vi "Initialization VI.vi"(8 "error in (no error)":errorcluster, 10 "Custom XML":string, 11 "Device Item Ref in":T1 format="%.0x") -> (0 "error out":errorcluster, 3 "Device Item Ref out":T1 format="%.0x")   [LabVIEW 2016, in "DMM-SWITCH-ScanList System Explorer.lvlib"]
uses:
  DMM-SWITCH-ScanList System Explorer.lvlib
  <vilib>/NI Veristand/Custom Device API/Custom Device Item Ref.ctl
  <instrlib>/niDMM/nidmm.llb/niDMM Function.ctl
  <instrlib>/niDMM/nidmm.llb/niDMM Resolution in Digits.ctl
  <instrlib>/niSwitch/niSwitch.llb/niSwitch Topologies.ctl
  <instrlib>/niSwitch/niSwitch.llb/niSwitch Trigger Input.ctl
  <instrlib>/niSwitch/niSwitch.llb/niSwitch Scan Advanced Output.ctl
  <instrlib>/niDMM/nidmm.llb/niDMM Measurement Complete.ctl
  <instrlib>/niDMM/nidmm.llb/niDMM Trigger.ctl
  Pages/Configuration Controls/DMM Temp.ctl
  <instrlib>/niDMM/nidmm.llb/niDMM Transducer Type.ctl
  <instrlib>/niDMM/nidmm.llb/niDMM Thermocouple Type.ctl
  <instrlib>/niDMM/nidmm.llb/niDMM RTD Type.ctl
  <instrlib>/niDMM/nidmm.llb/niDMM Thermistor Type.ctl
  <vilib>/NI Veristand/Custom Device API/Custom Device Channel.ctl
  <vilib>/NI Veristand/Custom Device API/Custom Device Channel Type.ctl
  Shared/Constants.vi
  <vilib>/NI Veristand/Custom Device API/Custom Device API.lvlib
  Shared/DMM-SWITCH-ScanList Shared.lvlib
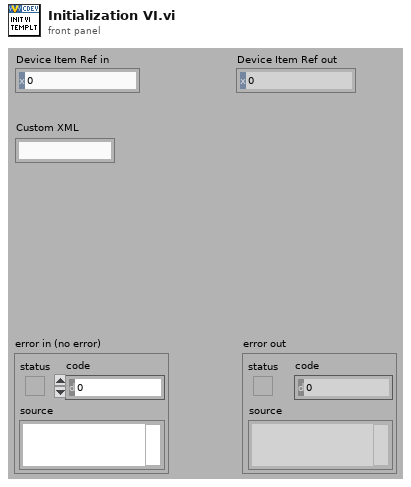
[diagram p1: front panel]
types:
  T1 = typedef "Custom Device API.lvlib/Custom Device Item Ref.ctl" = u64
  T2 = typedef "DMM-SWITCH-ScanList System Explorer.lvlib/DMM Temp.ctl" = cluster{"DMM Temp - Transducer Type":T3, "DMM Temp - Thermocouple Type":T4, "DMM Temp - Fixed Reference Junction":dbl, "DMM Temp - RTD Type":T5, "DMM Temp - RTD Resistance":dbl, "DMM Temp - Thermistor Type":T6, "DMM Temp - RTD A":dbl, "DMM Temp - RTD B":dbl, "DMM Temp - RTD C":dbl, "DMM Temp - Thermistor A":dbl, "DMM Temp - Thermistor B":dbl, "DMM Temp - Thermistor C":dbl}
  T3 = typedef "niDMM Transducer Type.ctl" = i32
  T4 = typedef "niDMM Thermocouple Type.ctl" = i32
  T5 = typedef "niDMM RTD Type.ctl" = enum16{"Custom", "Pt3750", "Pt3851", "Pt3911", "Pt3916", "Pt3920", "Pt3928"}
  T6 = typedef "niDMM Thermistor Type.ctl" = enum16{"Custom", "44004", "44006", "44007"}
  T7 = typedef "niDMM Trigger.ctl" = enum16{"Immediate", "External", "TTL 0", "TTL 1", "TTL 2", "TTL 3", "TTL 4", "TTL 5", "TTL 6", "Software", "TTL 7", "PXI Star", "LBR Trig 1", "Aux Trig 1"}
  T8 = typedef "niDMM Measurement Complete.ctl" = enum16{"None", "External", "TTL 0", "TTL 1", "TTL 2", "TTL 3", "TTL 4", "TTL 5", "TTL 6", "TTL 7", "LBR Trig 0"}
  T9 = typedef "niSwitch Scan Advanced Output.ctl" = enum16{"None", "External", "TTL0", "TTL1", "TTL2", "TTL3", "TTL4", "TTL5", "TTL6", "TTL7", "ECL0", "ECL1", "PXI Star", "Rear Connector", "Front Connector", "Rear Connector Module 1", "Rear Connector Module 2", "Rear Connector Module 3", "Rear Connector Module 4", "Rear Connector Module 5", "Rear Connector Module 6", "Rear Connector Module 7", "Rear Connector Module 8", "Rear Connector Module 9", "Rear Connector Module 10", "Rear Connector Module 11", "Rear Connector Module 12", "Front Connector Module 1", "Front Connector Module 2", "Front Connector Module 3", "Front Connector Module 4", "Front Connector Module 5", "Front Connector Module 6", "Front Connector Module 7", "Front Connector Module 8", "Front Connector Module 9", "Front Connector Module 10", "Front Connector Module 11", "Front Connector Module 12"}
  T10 = typedef "niSwitch Trigger Input.ctl" = enum16{"Immediate", "External", "TTL0", "TTL1", "TTL2", "TTL3", "TTL4", "TTL5", "TTL6", "TTL7", "ECL0", "ECL1", "PXI Star", "Software Trigger Function", "Rear Connector", "Front Connector", "Rear Connector of Module 1", "Rear Connector of Module 2", "Rear Connector of Module 3", "Rear Connector of Module 4", "Rear Connector of Module 5", "Rear Connector of Module 6", "Rear Connector of Module 7", "Rear Connector of Module 8", "Rear Connector of Module 9", "Rear Connector of Module 10", "Rear Connector of Module 11", "Rear Connector of Module 12", "Front Connector of Module 1", "Front Connector of Module 2", "Front Connector of Module 3", "Front Connector of Module 4", "Front Connector of Module 5", "Front Connector of Module 6", "Front Connector of Module 7", "Front Connector of Module 8", "Front Connector of Module 9", "Front Connector of Module 10", "Front Connector of Module 11", "Front Connector of Module 12"}
  T11 = typedef "niDMM Function.ctl" = enum16{"DC Volts", "AC Volts", "DC Current", "AC Current", "2-wire Resistance", "4-wire Resistance", "Diode", "Frequency", "Period", "AC Volts DC Coupled", "Capacitance", "Inductance", "Temperature"}
  T12 = typedef "niSwitch Topologies.ctl" = string
  T13 = typedef "niDMM Resolution in Digits.ctl" = dbl
  T14 = typedef "Custom Device API.lvlib/Custom Device Channel.ctl" = cluster{"Type":T15, "Units":string, "Default Value":dbl, "Faultable":bool, "Scalable":bool}
  T15 = typedef "Custom Device API.lvlib/Custom Device Channel Type.ctl" = enum16{"Input", "Output"}
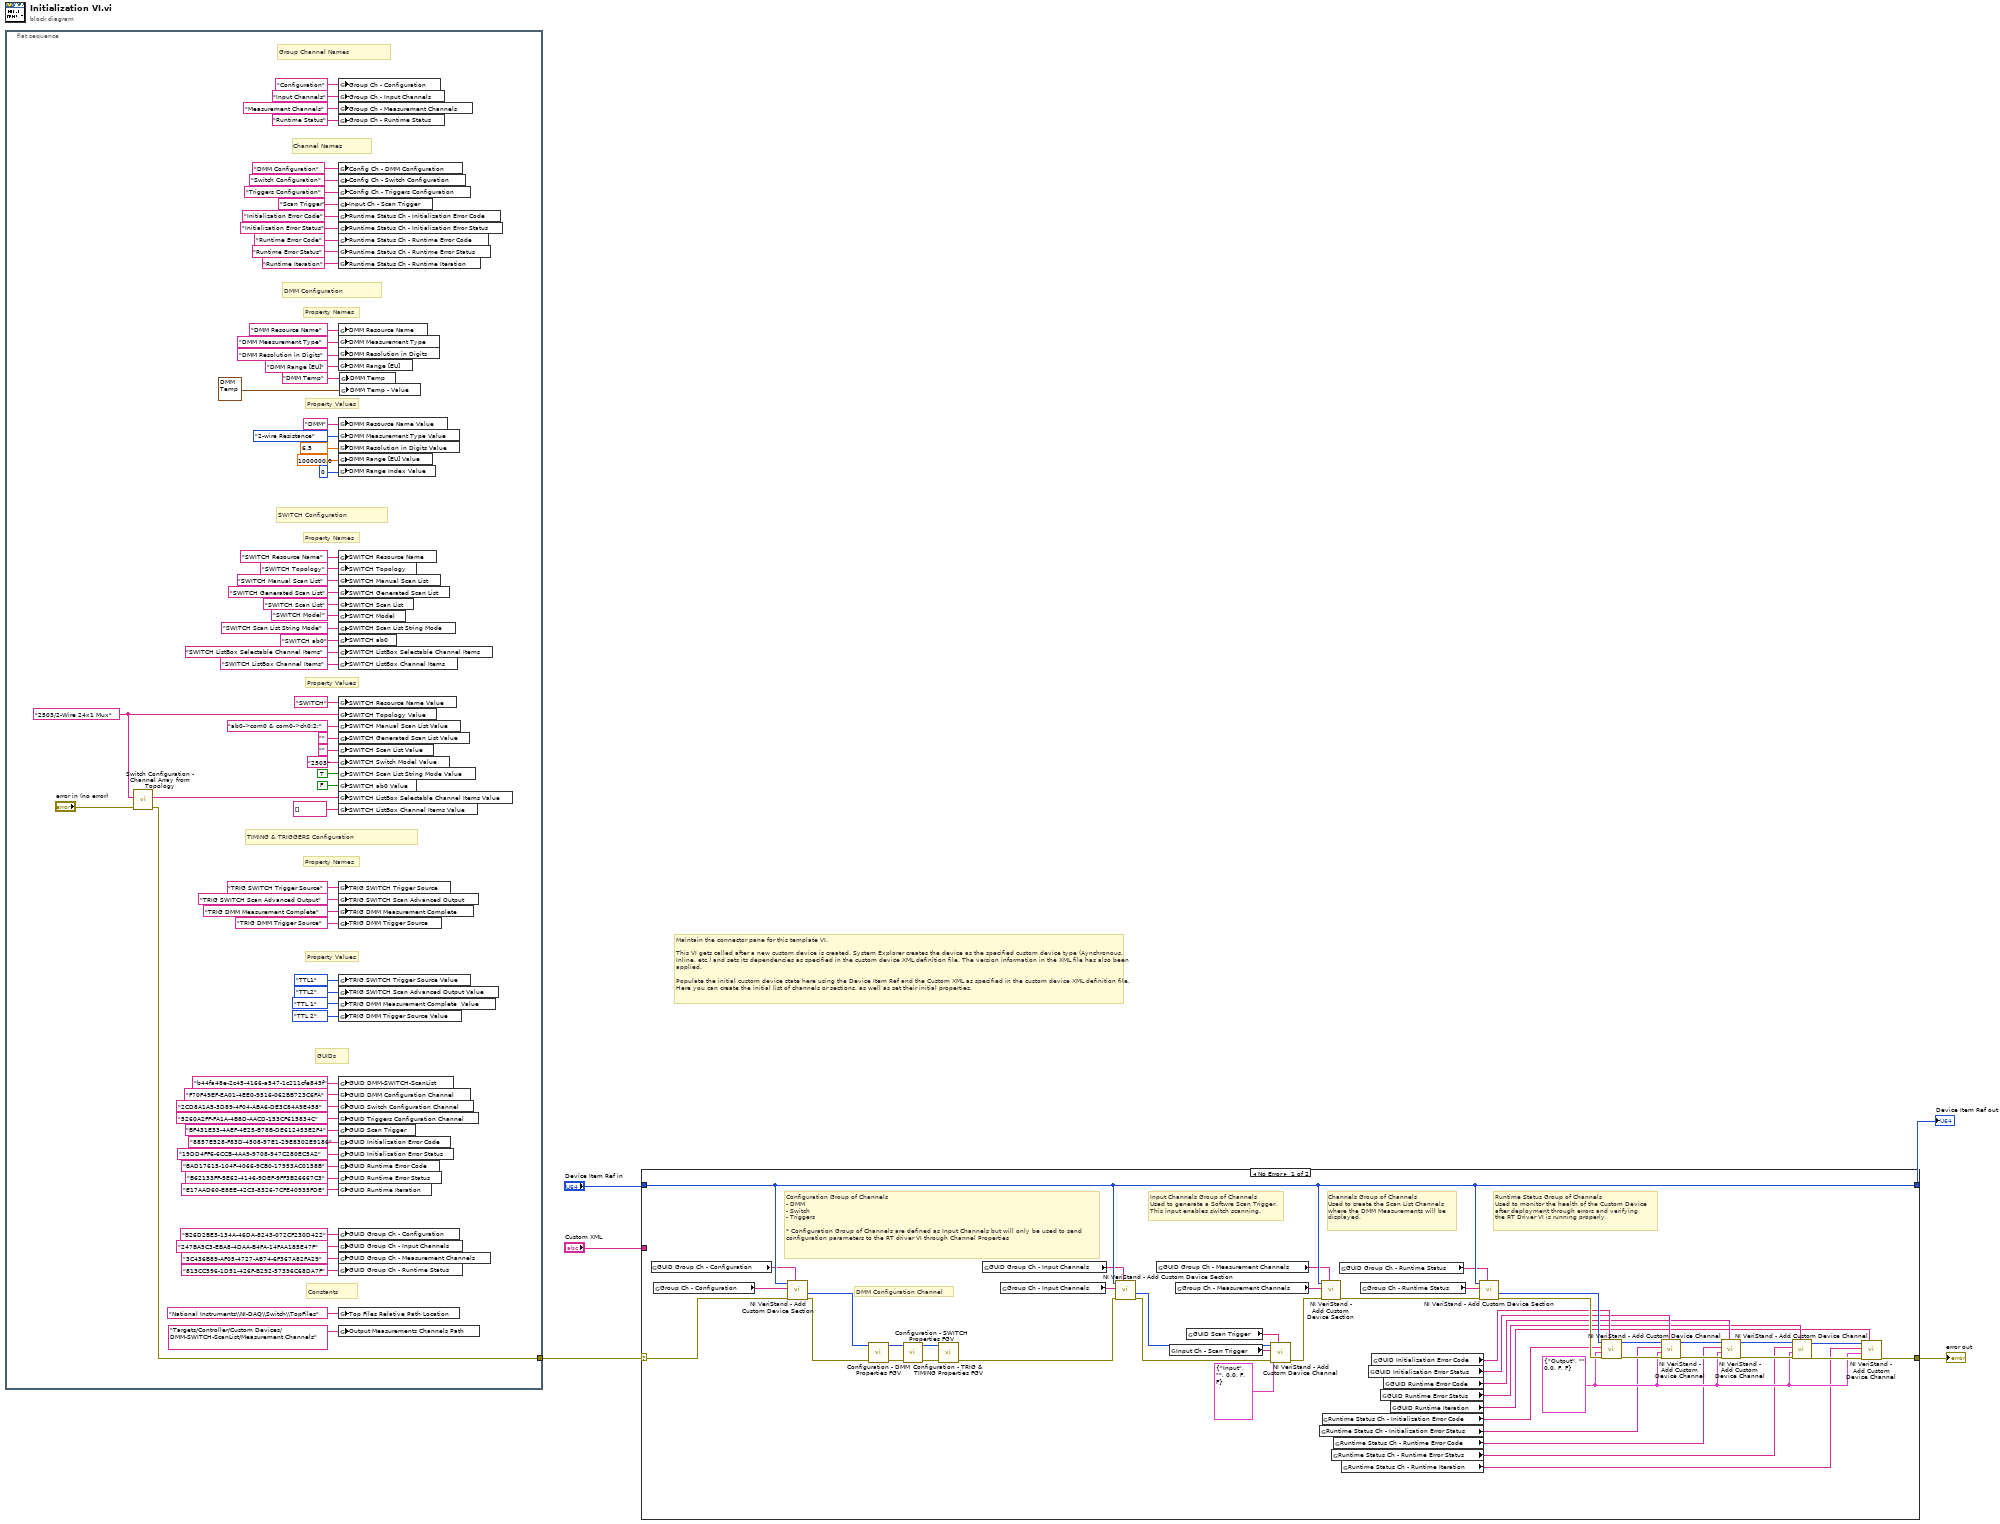
[diagram p0: block diagram]
diagram:
  # "Maintain the connector pane for this template VI.\n\nThis VI gets called after a new custom device is created. System Explorer creates the device as the specified custom device type (Aynchronous, Inline, etc.) and sets its dependencies as specified in the custom device XML definition file. The version information in the XML file has also been applied.\n\nPopulate the initial custom device state here using the Device Item Ref and the Custom XML as specified in the custom device XML definition file. Here you can create the initial list of channels or sections, as well as set their initial properties."
  n1 = flat-sequence {
    tunnel: [w56] -> w5
    frame #0 {
      w57 = T12 "2503/2-Wire 24x1 Mux" ("SWITCH Topology")
      w73 = T13 6.5 items=["3 1/2"=3.5, "4 1/2"=4.5, "5 1/2"=5.5, "6 1/2"=6.5, "7 1/2"=7.5] ("Resolution in Digits")
      # "Channel Names"
      # "Group Channel Names"
      # "Property Values"
      # "Property Names"
      # "Property Values"
      # "Property Names"
      # "Property Values"
      # "Property Names"
      # "Constants"
      # "DMM Configuration"
      # "GUIDs"
      # "TIMING & TRIGGERS Configuration"
      # "SWITCH Configuration"
      n2 = call "Switch Configuration - Channel Array from Topology.vi"("error in (no error)"="error in (no error)", "Selected Mux Topology"=w57) -> ("error out"=w56:errorcluster, "Channel Array Out"=w55:string[])  [unwired: 8 in]
      n3 = global write "Constants.vi" "Group Ch - Configuration"("Configuration" ("Group Ch - Configuration")) -> ()
      n4 = global write "Constants.vi" "Group Ch - Input Channels"("Input Channels" ("Group Ch - Input Channels")) -> ()
      n5 = global write "Constants.vi" "Group Ch - Measurement Channels"("Measurement Channels" ("Group Ch - Measurement Channels")) -> ()
      n6 = global write "Constants.vi" "Group Ch - Runtime Status"("Runtime Status" ("Group Ch - Runtime Status")) -> ()
      n7 = global write "Constants.vi" "Config Ch - DMM Configuration"("DMM Configuration" ("Group Ch - Configuration")) -> ()
      n8 = global write "Constants.vi" "Config Ch - Switch Configuration"("Switch Configuration" ("Group Ch - Input Channels")) -> ()
      n9 = global write "Constants.vi" "Config Ch - Triggers Configuration"("Triggers Configuration" ("Group Ch - Measurement Channels")) -> ()
      n10 = global write "Constants.vi" "Input Ch - Scan Trigger"("Scan Trigger" ("Group Ch - Runtime Status")) -> ()
      n11 = global write "Constants.vi" "Runtime Status Ch - Initialization Error Code"("Initialization Error Code" ("Group Ch - Configuration")) -> ()
      n12 = global write "Constants.vi" "Runtime Status Ch - Initialization Error Status"("Initialization Error Status" ("Group Ch - Input Channels")) -> ()
      n13 = global write "Constants.vi" "Runtime Status Ch - Runtime Error Code"("Runtime Error Code" ("Group Ch - Measurement Channels")) -> ()
      n14 = global write "Constants.vi" "Runtime Status Ch - Runtime Error Status"("Runtime Error Status" ("Group Ch - Runtime Status")) -> ()
      n15 = global write "Constants.vi" "Runtime Status Ch - Runtime Iteration"("Runtime Iteration" ("Group Ch - Runtime Status")) -> ()
      n16 = global write "Constants.vi" "DMM Resource Name"("DMM Resource Name" ("DMM Resource Name")) -> ()
      n17 = global write "Constants.vi" "DMM Measurement Type"("DMM Measurement Type" ("DMM Measurement Type")) -> ()
      n18 = global write "Constants.vi" "DMM Resolution in Digits"("DMM Resolution in Digits" ("DMM Resolution in Digits")) -> ()
      n19 = global write "Constants.vi" "DMM Range [EU]"("DMM Range [EU]" ("DMM Range [EU]")) -> ()
      n20 = global write "Constants.vi" "DMM Resource Name Value"("DMM" ("Value")) -> ()
      n21 = global write "Constants.vi" "DMM Measurement Type Value"(niDMM_Function."2-wire Resistance" ("Function")) -> ()
      n22 = global write "Constants.vi" "DMM Resolution in Digits Value"(w73) -> ()
      n23 = global write "Constants.vi" "DMM Range [EU] Value"(1000000.0 ("DMM Range [EU] Value")) -> ()
      n24 = global write "Constants.vi" "DMM Range Index Value"(u16 0 ("DMM Range Index")) -> ()
      n25 = global write "Constants.vi" "SWITCH Resource Name"("SWITCH Resource Name" ("SWITCH Resource Name")) -> ()
      n26 = global write "Constants.vi" "SWITCH Topology"("SWITCH Topology" ("SWITCH Topology")) -> ()
      n27 = global write "Constants.vi" "SWITCH Manual Scan List"("SWITCH Manual Scan List" ("SWITCH Manual Scan List")) -> ()
      n28 = global write "Constants.vi" "SWITCH Generated Scan List"("SWITCH Generated Scan List" ("SWITCH Generated Scan List")) -> ()
      n29 = global write "Constants.vi" "SWITCH Scan List"("SWITCH Scan List" ("SWITCH Scan List")) -> ()
      n30 = global write "Constants.vi" "SWITCH Model"("SWITCH Model" ("SWITCH Switch Model")) -> ()
      n31 = global write "Constants.vi" "SWITCH Scan List String Mode"("SWITCH Scan List String Mode" ("SWITCH Scan List String Mode")) -> ()
      n32 = global write "Constants.vi" "SWITCH ab0"("SWITCH ab0" ("SWITCH ab0")) -> ()
      n33 = global write "Constants.vi" "SWITCH ListBox Selectable Channel Items"("SWITCH ListBox Selectable Channel Items" ("SWITCH ListBox Selectable Channel Items")) -> ()
      n34 = global write "Constants.vi" "SWITCH ListBox Channel Items"("SWITCH ListBox Channel Items" ("SWITCH ListBox Channel Items")) -> ()
      n35 = global write "Constants.vi" "SWITCH Resource Name Value"("SWITCH" ("SWITCH Resource Name")) -> ()
      n36 = global write "Constants.vi" "SWITCH Topology Value"(w57) -> ()
      n37 = global write "Constants.vi" "SWITCH Manual Scan List Value"("ab0->com0 & com0->ch0:2;" ("SWITCH Manual Scan List")) -> ()
      n38 = global write "Constants.vi" "SWITCH Generated Scan List Value"("" ("SWITCH Generated Scan List")) -> ()
      n39 = global write "Constants.vi" "SWITCH Scan List Value"("" ("SWITCH Scan List")) -> ()
      n40 = global write "Constants.vi" "SWITCH Switch Model Value"("2503" ("SWITCH Switch Model")) -> ()
      n41 = global write "Constants.vi" "SWITCH Scan List String Mode Value"(TRUE ("SWITCH Scan List String Mode")) -> ()
      n42 = global write "Constants.vi" "SWITCH ab0 Value"(FALSE ("SWITCH ab0")) -> ()
      n43 = global write "Constants.vi" "SWITCH ListBox Selectable Channel Items Value"(w55) -> ()
      n44 = global write "Constants.vi" "SWITCH ListBox Channel Items Value"(string[] [] ("SWITCH ListBox Channel Items")) -> ()
      n45 = global write "Constants.vi" "TRIG SWITCH Trigger Source"("TRIG SWITCH Trigger Source" ("TRIG SWITCH Trigger Source")) -> ()
      n46 = global write "Constants.vi" "TRIG SWITCH Scan Advanced Output"("TRIG SWITCH Scan Advanced Output" ("TRIG SWITCH Scan Advanced Output")) -> ()
      n47 = global write "Constants.vi" "TRIG DMM Measurement Complete"("TRIG DMM Measurement Complete" ("TRIG DMM Measurement Complete")) -> ()
      n48 = global write "Constants.vi" "TRIG DMM Trigger Source"("TRIG DMM Trigger Source" ("TRIG DMM Trigger Source")) -> ()
      n49 = global write "Constants.vi" "TRIG SWITCH Trigger Source Value"(niSwitch_Trigger_Input."TTL1" ("TRIG SWITCH Trigger Source")) -> ()
      n50 = global write "Constants.vi" "TRIG SWITCH Scan Advanced Output Value"(niSwitch_Scan_Advanced_Output."TTL2" ("TRIG SWITCH Scan \nAdvanced Output")) -> ()
      n51 = global write "Constants.vi" "TRIG DMM Measurement Complete  Value"(niDMM_Measurement_Complete."TTL 1" ("TRIG DMM Measurement \nComplete Destination")) -> ()
      n52 = global write "Constants.vi" "TRIG DMM Trigger Source Value"(niDMM_Trigger."TTL 2" ("TRIG DMM Trigger Source")) -> ()
      n53 = global write "Constants.vi" "GUID DMM-SWITCH-ScanList"("b44fa48e-2c45-4166-a547-1c211cfe843f" ("GUID DMM-SWITCH-ScanList")) -> ()
      n54 = global write "Constants.vi" "GUID DMM Configuration Channel"("F70F49EF-EA01-4EE0-9516-062BB723C6FA" ("GUID DMM Configuration Channel")) -> ()
      n55 = global write "Constants.vi" "GUID Switch Configuration Channel"("2CD8A1A5-3D89-4F04-ABA6-DE3C84A9E458" ("GUID Switch Configuration Channel")) -> ()
      n56 = global write "Constants.vi" "GUID Triggers Configuration Channel"("5260A2FF-FA1A-4B8D-AACD-153CF615834C" ("GUID Triggers Configuration Channel")) -> ()
      n57 = global write "Constants.vi" "GUID Scan Trigger"("BF431E33-4AEF-4E25-B78B-DE612453E2F4" ("GUID DMM-SWITCH-ScanList")) -> ()
      n58 = global write "Constants.vi" "GUID Initialization Error Code"("8857E528-F83D-4508-97E1-29E8302E9186" ("GUID DMM Configuration Channel")) -> ()
      n59 = global write "Constants.vi" "GUID Initialization Error Status"("19DD4FF6-6CCB-4AA9-9708-947C280EC5A2" ("GUID Switch Configuration Channel")) -> ()
      n60 = global write "Constants.vi" "GUID Runtime Error Code"("BAD17615-104F-4066-9CB0-17953AC0158B" ("GUID Triggers Configuration Channel")) -> ()
      n61 = global write "Constants.vi" "GUID Runtime Error Status"("B62133FF-5E62-4146-9DEF-9FF3B26667C3" ("GUID Triggers Configuration Channel")) -> ()
      n62 = global write "Constants.vi" "GUID Runtime Iteration"("E17AAD60-E8EE-42C3-8326-7CFE40935FDE" ("GUID Triggers Configuration Channel")) -> ()
      n63 = global write "Constants.vi" "GUID Group Ch - Configuration"("B26D2BE3-134A-46DA-8243-072CF230D422" ("GUID Triggers Configuration Channel")) -> ()
      n64 = global write "Constants.vi" "GUID Group Ch - Input Channels"("247BA5C3-EBA8-4DAA-B4FA-14FAA185E47F" ("GUID Triggers Configuration Channel")) -> ()
      n65 = global write "Constants.vi" "GUID Group Ch - Measurement Channels"("3C436B89-AF05-4727-AB74-6F367A82FA29" ("GUID Triggers Configuration Channel")) -> ()
      n66 = global write "Constants.vi" "GUID Group Ch - Runtime Status"("813CC596-1D51-426F-B292-57396C68DA7F" ("GUID Triggers Configuration Channel")) -> ()
      n67 = global write "Constants.vi" "Top Files Relative Path Location"("National Instruments\\NI-DAQ\\Switch\\TopFiles" ("Top Files Relative Path Location")) -> ()
      n68 = global write "Constants.vi" "Output Measurements Channels Path"("Targets/Controller/Custom Devices/DMM-SWITCH-ScanList/Measurement Channels" ("Output Measurements Channels Path")) -> ()
      n69 = global write "Constants.vi" "DMM Temp"("DMM Temp" ("DMM Temp")) -> ()
      n70 = global write "Constants.vi" "DMM Temp - Value"(T2 {"DMM Temp - Transducer Type"=1, "DMM Temp - Thermocouple Type"=6, "DMM Temp - Fixed Reference Junction"=25.0, "DMM Temp - RTD Type"=enum."Pt3851", "DMM Temp - RTD Resistance"=100.0, "DMM Temp - Thermistor Type"=enum."44006", "DMM Temp - RTD A"=0.0039083, "DMM Temp - RTD B"=-5.775e-07, "DMM Temp - RTD C"=-4.183e-12, "DMM Temp - Thermistor A"=0.0010295, "DMM Temp - Thermistor B"=0.0002391, "DMM Temp - Thermistor C"=1.568e-07} ("DMM Temp - Value")) -> ()
    }
  }
  n71 = case shown="No Error" w5 {
    selector: w5 -> [w117 w123]
    tunnel: [w93 w123] -> w1
    tunnel: [w98 w122] -> w3
    tunnel: "Device Item Ref in" -> [w98 w122]
    tunnel: "Custom XML" -> [_ _]
    frame No Error {
      w104 = T14 {"Type"=enum."Output", "Units"="", "Default Value"=0.0, "Faultable"=FALSE, "Scalable"=FALSE} ("Channel")
      # "Input Channels Group of Channels\nUsed to generate a Softwre Scan Trigger.\nThis input enables switch scanning."
      # "Runtime Status Group of Channels\nUsed to monitor the health of the Custom Device\nafter deployment through errors and verifying \nthe RT Driver VI is running properly."
      # "Channels Group of Channels\nUsed to create the Scan List Channels\nwhere the DMM Measurements will be\ndisplayed."
      # "DMM Configuration Channel"
      # "Configuration Group of Channels\n- DMM\n- Switch\n- Triggers\n\n* Configuration Group of Channels are defined as Input Channels but will only be used to send \nconfiguration parameters to the RT driver VI through Channel Properties"
      n72 = global read "Constants.vi" "GUID Group Ch - Configuration"() -> (w85:string)
      n73 = global read "Constants.vi" "Group Ch - Configuration"() -> (w86:string)
      n74 = call <vilib>:"NI VeriStand - Add Custom Device Section.vi"("GUID (Default Section)"=w85, "error in (no error)"=w117, "Section Name"=w86, "Parent Ref in"=w98) -> ("error out"=w121:errorcluster, "Section Ptr"=w120:T1)  [unwired: 4 in, 2 out]
      n75 = call "Configuration - DMM Properties FGV.vi"("error in (no error)"=w121, "Configuration Group of Channels Ref In"=w120) -> ("error out"=w116:errorcluster, "Configuration Group of Channels Ref Out"=w119:T1)  [unwired: 8 in]
      n76 = call "Configuration - SWITCH Properties FGV.vi"("error in (no error)"=w116, "Parent Ref in"=w119) -> ("error out"=w115:errorcluster, "Parent Ref out"=w118:T1)  [unwired: 8 in]
      n77 = call "Configuration - TRIG & TIMING Properties FGV.vi"("error in (no error)"=w115, "Parent Ref in"=w118) -> ("error out"=w100:errorcluster)  [unwired: 9 in]
      n78 = global read "Constants.vi" "GUID Group Ch - Input Channels"() -> (w84:string)
      n79 = global read "Constants.vi" "Group Ch - Input Channels"() -> (w96:string)
      n80 = call <vilib>:"NI VeriStand - Add Custom Device Section.vi"("GUID (Default Section)"=w84, "error in (no error)"=w100, "Section Name"=w96, "Parent Ref in"=w98) -> ("error out"=w102:errorcluster, "Section Ptr"=w103:T1)  [unwired: 4 in, 2 out]
      n81 = global read "Constants.vi" "GUID Group Ch - Measurement Channels"() -> (w83:string)
      n82 = global read "Constants.vi" "Input Ch - Scan Trigger"() -> (w92:string)
      n83 = global read "Constants.vi" "Group Ch - Measurement Channels"() -> (w95:string)
      n84 = global read "Constants.vi" "GUID Scan Trigger"() -> (w76:string)
      n85 = call <vilib>:"NI VeriStand - Add Custom Device Channel.vi"("GUID (Default Channel)"=w76, "error in (no error)"=w102, "Channel"=T14 {"Type"=enum."Input", "Units"="", "Default Value"=0.0, "Faultable"=FALSE, "Scalable"=FALSE}, "Channel Name"=w92, "Parent Ref in"=w103) -> ("error out"=w101:errorcluster)  [unwired: 3 in, 3 out]
      n86 = global read "Constants.vi" "Runtime Status Ch - Initialization Error Status"() -> (w90:string)
      n87 = call <vilib>:"NI VeriStand - Add Custom Device Section.vi"("GUID (Default Section)"=w83, "error in (no error)"=w101, "Section Name"=w95, "Parent Ref in"=w98) -> ("error out"=w114:errorcluster)  [unwired: 4 in, 3 out]
      n88 = global read "Constants.vi" "Runtime Status Ch - Initialization Error Code"() -> (w91:string)
      n89 = global read "Constants.vi" "Runtime Status Ch - Runtime Error Status"() -> (w88:string)
      n90 = global read "Constants.vi" "Runtime Status Ch - Runtime Error Code"() -> (w89:string)
      n91 = global read "Constants.vi" "GUID Group Ch - Runtime Status"() -> (w82:string)
      n92 = global read "Constants.vi" "Runtime Status Ch - Runtime Iteration"() -> (w87:string)
      n93 = global read "Constants.vi" "Group Ch - Runtime Status"() -> (w94:string)
      n94 = global read "Constants.vi" "GUID Initialization Error Status"() -> (w80:string)
      n95 = global read "Constants.vi" "GUID Initialization Error Code"() -> (w81:string)
      n96 = global read "Constants.vi" "GUID Runtime Error Status"() -> (w78:string)
      n97 = global read "Constants.vi" "GUID Runtime Error Code"() -> (w79:string)
      n98 = global read "Constants.vi" "GUID Runtime Iteration"() -> (w77:string)
      n99 = call <vilib>:"NI VeriStand - Add Custom Device Section.vi"("GUID (Default Section)"=w82, "error in (no error)"=w114, "Section Name"=w94, "Parent Ref in"=w98) -> ("error out"=w106:errorcluster, "Section Ptr"=w105:T1)  [unwired: 4 in, 2 out]
      n100 = call <vilib>:"NI VeriStand - Add Custom Device Channel.vi"("GUID (Default Channel)"=w81, "error in (no error)"=w106, "Channel"=w104, "Channel Name"=w91, "Parent Ref in"=w105) -> ("error out"=w113:errorcluster, "Parent Ref out"=w97:T1)  [unwired: 3 in, 2 out]
      n101 = call <vilib>:"NI VeriStand - Add Custom Device Channel.vi"("GUID (Default Channel)"=w80, "error in (no error)"=w113, "Channel"=w104, "Channel Name"=w90, "Parent Ref in"=w97) -> ("error out"=w111:errorcluster, "Parent Ref out"=w112:T1)  [unwired: 3 in, 2 out]
      n102 = call <vilib>:"NI VeriStand - Add Custom Device Channel.vi"("GUID (Default Channel)"=w79, "error in (no error)"=w111, "Channel"=w104, "Channel Name"=w89, "Parent Ref in"=w112) -> ("error out"=w109:errorcluster, "Parent Ref out"=w110:T1)  [unwired: 3 in, 2 out]
      n103 = call <vilib>:"NI VeriStand - Add Custom Device Channel.vi"("GUID (Default Channel)"=w78, "error in (no error)"=w109, "Channel"=w104, "Channel Name"=w88, "Parent Ref in"=w110) -> ("error out"=w108:errorcluster, "Parent Ref out"=w107:T1)  [unwired: 3 in, 2 out]
      n104 = call <vilib>:"NI VeriStand - Add Custom Device Channel.vi"("GUID (Default Channel)"=w77, "error in (no error)"=w108, "Channel"=w104, "Channel Name"=w87, "Parent Ref in"=w107) -> ("error out"=w93:errorcluster)  [unwired: 3 in, 3 out]
    }
    frame Error {
    }
  }
  "error out" <- w1
  "Device Item Ref out" <- w3
